vi "Scale Channel.vi"(9 "channel to scale":i32, 10 "Waveform in":waveform(dbl), 11 "Channel Settings":T1[](array[typedef])) -> (2 "Scaled waveform":waveform(dbl))   [LabVIEW 2021, in "Acquisition.lvlib"]
doc: "Use the index 'channel to scale' to apply the calibration coefficients from the corresponding channel in 'Channel Settings' to 'Waveform in' and return 'Scaled waveform'."
uses:
  Acquisition.lvlib
  Channel Settings.ctl
  IO Device.ctl
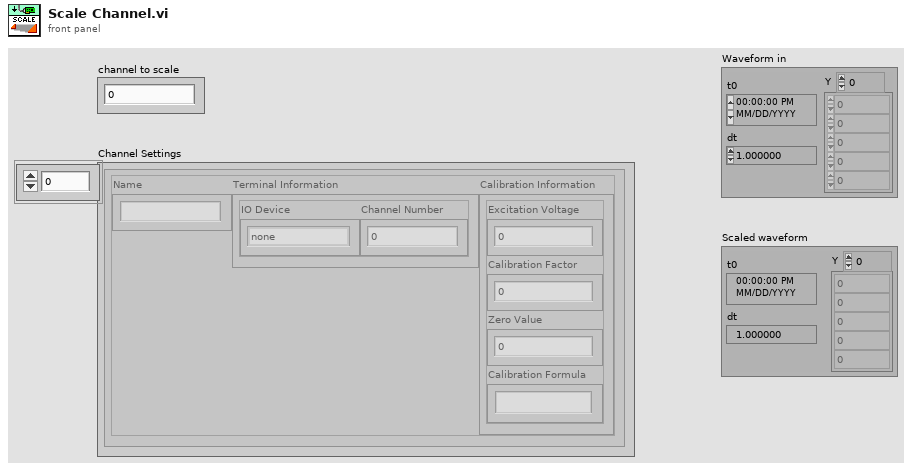
[diagram p1: front panel]
types:
  T1 = typedef "Acquisition.lvlib/Channel Settings.ctl" = cluster{"Name":string, "Terminal Information":cluster{"IO Device":T2, "Channel Number":i32}, "Calibration Information":cluster{"Excitation Voltage":dbl, "Calibration Factor":dbl, "Zero Value":dbl, "Calibration Formula":string}}
  T2 = typedef "Acquisition.lvlib/IO Device.ctl" = enum16{"none", "9219", "9401"}
  T3 = cluster{"Excitation Voltage":dbl, "Calibration Factor":dbl, "Zero Value":dbl, "Calibration Formula":string}
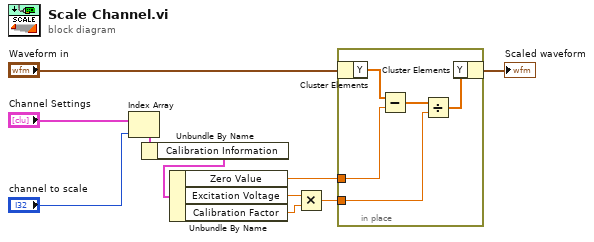
[diagram p0: block diagram]
diagram:
  n1 = Index Array(array="Channel Settings", index="channel to scale") -> (element=w5:T1)
  n2 = Unbundle By Name(w5) -> ("Calibration Information"=w6:T3)
  n3 = Unbundle By Name(w6) -> ("Zero Value"=w10:dbl, "Excitation Voltage"=w7:dbl, "Calibration Factor"=w8:dbl)
  n4 = Multiply(x=w7, y=w8) -> (x*y=w9:dbl)
  n5 = in-place {
    in-place-border: w9 -> [w12]
    in-place-border: w10 -> [w14]
    n6 = in-place-cluster #1("Waveform in") -> ("Y"=w15:dbl[])
    n7 = Subtract(x=w15, y=w14) -> (x-y=w13:dbl[])
    n8 = Divide(x=w13, y=w12) -> (x/y=w11:dbl[])
    n9 = in-place-cluster #1("Y"=w11) -> (→"Scaled waveform":waveform(dbl))
  }
